vi "Compile CHM.vi"(8 "error in (no error)":errorcluster, 11 "CHM Generator in":refnum<class "CHM Generator.lvclass">) -> (0 "error out":errorcluster, 2 "standard output":string, 3 "CHM Generator out":refnum<class "CHM Generator.lvclass">)   [LabVIEW 2027, in "CHM Generator.lvclass"]
uses:
  CHM Generator.lvclass
  <vilib>/Utility/sysdir.llb/System Directory Type.ctl
  CHM Generator.lvclass/CHM Generator.ctl
  Keyed Value Tree/Keyed Value Tree.lvclass
panel:
  out "return code":i32
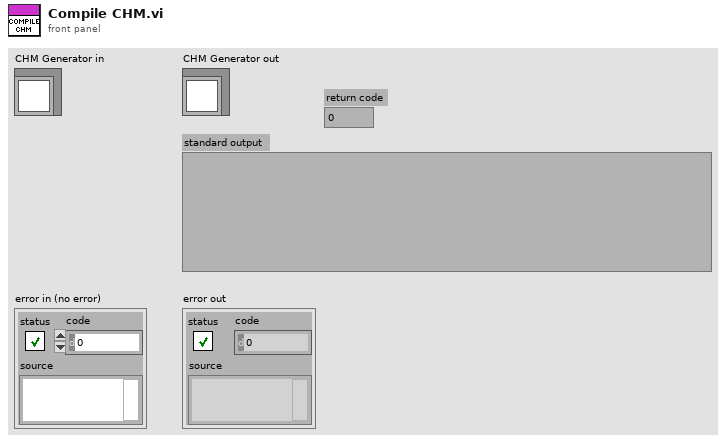
[diagram p1: front panel]
types:
  T1 = typedef "System Directory Type.ctl" = i32
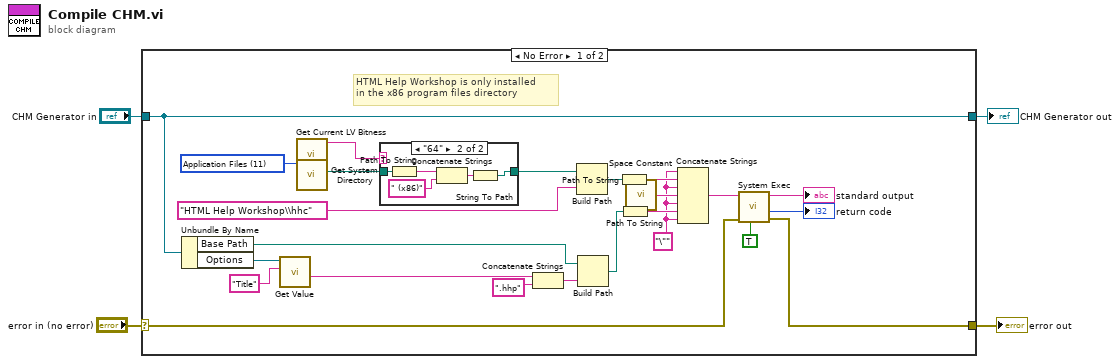
[diagram p0: block diagram]
diagram:
  n1 = case shown="No Error" "error in (no error)" {
    selector: "error in (no error)" -> [w9 w36]
    tunnel: [w8 w36] -> w3
    tunnel: [w28 w35] -> w1
    tunnel: "CHM Generator in" -> [w28 w35]
    frame No Error {
      w18 = "\"" ("string")
      w22 = T1 11 items=["User Home"=0, "User Desktop"=1, "User Documents"=2, "User Application Data"=3, "User Preferences"=4, "User Temporary"=5, "Public Documents"=6, "Public Application Data"=7, "Public Preferences"=8, "Public Cache"=13, "System Core Libraries"=9, "System Installed Libraries"=10, "Application Files"=11, "Boot Volume Root"=12] ("system directory type")
      # "HTML Help Workshop is only installed\nin the x86 program files directory"
      n2 = Unbundle By Name(w28) -> ("Base Path"=w12:path, "Options"=w17:refnum<class "Keyed Value Tree.lvclass">)
      n3 = call-dynamic "Get Value.vi"("name"="Title", "Keyed Value Tree in"=w17) -> ("value"=w15:string)  [unwired: 6 in, 3 out]
      n4 = call <vilib>:"Get Current LV Bitness.vi"() -> ("bitness"=w7:string)  [unwired: 11 in]
      n5 = call <vilib>:"Get System Directory.vi"("system directory type"=w22) -> ("system directory"=w6:path)  [unwired: 10 in]
      n6 = case shown="\"64\"" w7 {
        tunnel: w6 -> [w29 w34]
        tunnel: [w29 w30] -> w5
        frame "32", Default {
        }
        frame "64" {
          n7 = Path To String(path=w34) -> (string=w33:string)
          n8 = Concatenate Strings(w33, " (x86)" ("string")) -> (w31:string)
          n9 = String To Path(string=w31) -> (path=w30:path)
        }
      }
      n10 = Concatenate Strings(w15, ".hhp" ("string")) -> (w13:string)
      n11 = Build Path(base path=w5, name or relative path="HTML Help Workshop\\hhc") -> (appended path=w19:path)
      n12 = Build Path(base path=w12, name or relative path=w13) -> (appended path=w11:path)
      n13 = Path To String(path=w19) -> (string=w21:string)
      n14 = Path To String(path=w11) -> (string=w26:string)
      n15 = call <vilib>:"Space Constant.vi"() -> ("String"=w25:string)
      n16 = Concatenate Strings(w18, w21, w18, w25, w18, w26, w18) -> (w27:string)
      n17 = call <vilib>:"System Exec.vi"("run minimized? (F)"=TRUE, "error in (no error)"=w9, "command line"=w27) -> ("error out"=w8:errorcluster, "return code"=→"return code":i32, "standard output"=→"standard output":string)  [unwired: 5 in, 1 out]
    }
    frame Error {
    }
  }
  "error out" <- w3
  "CHM Generator out" <- w1
